vi "DepthImage Callback.vi"(4 "Depth Image Queue":refnum<queue>, 5 "Event Data":cluster{"sender":refnum<k24>, "e":refnum<k24>}, 6 "Control Ref":refnum<k24>, 7 "Event Common Data":T1) -> ()   [LabVIEW 2011]
uses:
  Microsoft.Kinect
  <vilib>/vision/Image Controls.llb/IMAQ Image.ctl
  Kinect Global Status.vi
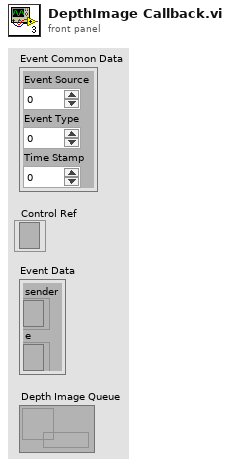
[diagram p1: front panel]
types:
  T1 = cluster{"Event Source":i32, "Event Type":u32, "Time Stamp":u32}
  T2 = typedef "Image Type" = u32
  T3 = typedef "IMAQ Image.ctl" = refnum<image>
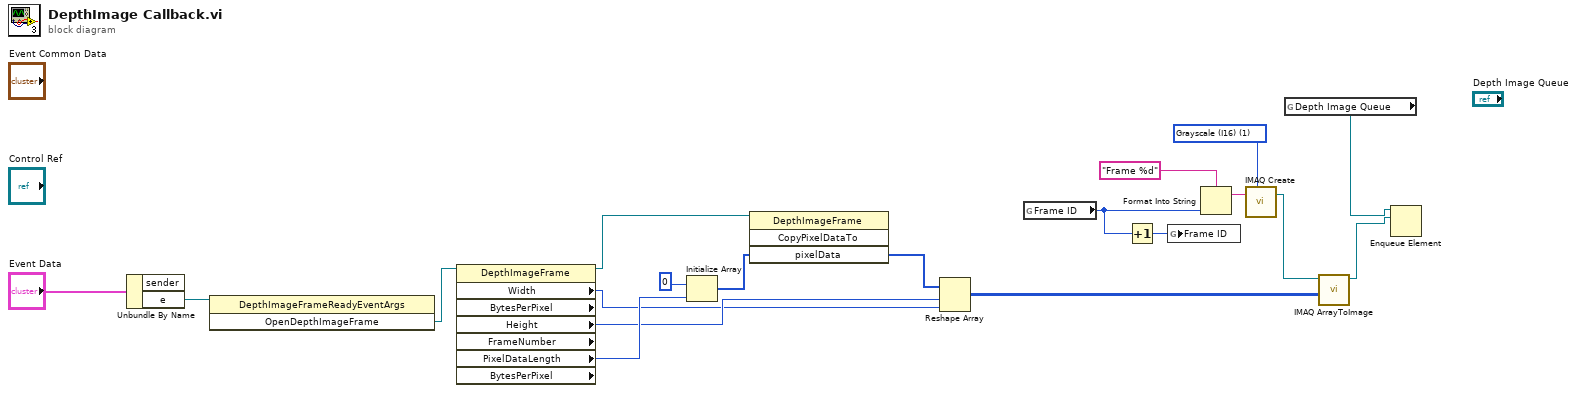
[diagram p0: block diagram]
diagram:
  w15 = T2 1 items=["Grayscale (U8)", "Grayscale (I16)", "Grayscale (SGL)", "Complex (CSG)", "RGB (U32)", "HSL (U32)", "RGB (U64)", "Grayscale (U16)"] ("Image Type")
  n1 = Unbundle By Name("Event Data") -> ("e"=w18:refnum<k24>)  [unwired: 1 out]
  n2 = invoke class="DepthImageFrameReadyEventArgs" method="OpenDepthImageFrame"(reference=w18) -> ("OpenDepthImageFrame"=w11:refnum<k24>)  [unwired: 2 in, 2 out]
  n3 = property on="Property Node" class="DepthImageFrame" props=["Width", "BytesPerPixel", "Height", "FrameNumber", "PixelDataLength", "BytesPerPixel"](reference=w11) -> (reference out=w10:refnum<k24>, "Width"=w9:i32, "Height"=w13:i32, "PixelDataLength"=w14:i32)  [unwired: 1 in, 4 out]
  n4 = Initialize Array(i16 0 ("element"), w14) -> (w8:i16[])
  n5 = invoke class="DepthImageFrame" method="CopyPixelDataTo"(reference=w10, "pixelData"=w8) -> ("pixelData"=w7:i16[])  [unwired: 2 in, 3 out]
  n6 = Reshape Array(w7, w13, w9) -> (w12:i16[][])
  n7 = global read "Kinect Global Status.vi" "Frame ID"() -> (w4:i32)
  n8 = Increment(x=w4) -> (x+1=w5:i32)
  n9 = global write "Kinect Global Status.vi" "Frame ID"(w5) -> ()
  n10 = Format Into String(format string="Frame %d" ("Image Name"), w4) -> (resulting string=w3:string)  [unwired: 2 in, 1 out]
  n11 = call "IMAQ Create"("Image Name"=w3, "Image Type"=w15) -> ("New Image"=w16:T3)  [unwired: 3 in, 1 out]
  n12 = global read "Kinect Global Status.vi" "Depth Image Queue"() -> (w2:refnum<queue>)
  n13 = call "IMAQ ArrayToImage"("Image Pixels (I16)"=w12, "Image"=w16) -> ("Image Out"=w1:T3)  [unwired: 8 in, 1 out]
  n14 = Enqueue Element(queue=w2, element=w1) -> ()  [unwired: 2 in, 3 out]
